vi "ConnectionTest.vi"() -> ()   [LabVIEW 2015]
uses:
  <vilib>/userdefined/High Color/IMAQdx.ctl
  <vilib>/vision/driver/IMAQdx.llb/IMAQdx Camera Control Mode.ctl
  <vilib>/vision/driver/IMAQdx.llb/IMAQdx Acquisition Mode.ctl
  <vilib>/vision/driver/IMAQdx.llb/IMAQdx Buffer Number Mode.ctl
  <vilib>/vision/driver/NI_Vision_Acquisition_Software.lvlib
panel:
  out "Image":T1(plugin-control)
  in  "Buffer Number Mode (Next)":T2
  in  "Number of Buffers":u32=1
  in  "Continuous?":T3
  out "error out":errorcluster
  in  "Camera Control Mode":T4
  in  "Session In":T5
  # "This is just me testing trying to connect the camera and LabView\n\nGenerally I will have a few programs titled testing where I am working on new things and then when they are complete or they have some functionality I go to Save As and do the thing where I rename the VI"
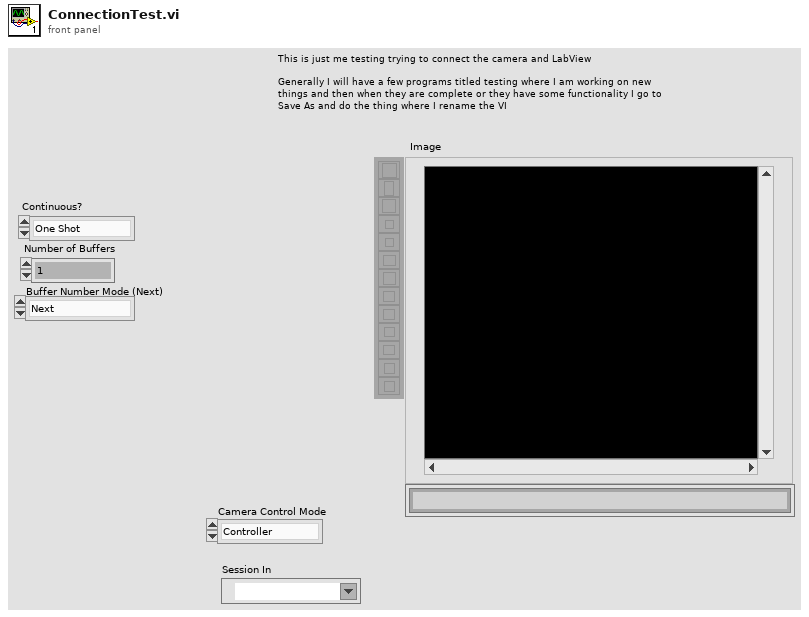
[diagram p1: front panel]
types:
  T1 = typedef "IMAQ Image.ctl" = refnum<image>
  T2 = typedef "NI_Vision_Acquisition_Software.lvlib/IMAQdx Buffer Number Mode.ctl" = enum32{"Next", "Last", "Buffer Number", "Every", "Last New"}
  T3 = typedef "NI_Vision_Acquisition_Software.lvlib/IMAQdx Acquisition Mode.ctl" = enum32{"One Shot", "Continuous"}
  T4 = typedef "NI_Vision_Acquisition_Software.lvlib/IMAQdx Camera Control Mode.ctl" = enum32{"Controller", "Listener"}
  T5 = typedef "IMAQdx.ctl" = refnum<k21>
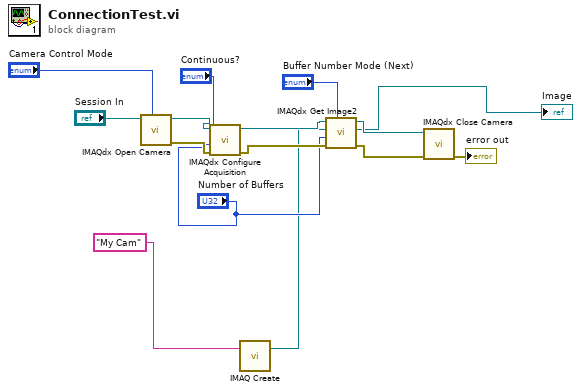
[diagram p0: block diagram]
diagram:
  n1 = call <vilib>:"IMAQdx Open Camera.vi"("Camera Control Mode"="Camera Control Mode", "Session In"="Session In") -> ("error out"=w11:errorcluster, "Session Out"=w12:T5)  [unwired: 8 in]
  n2 = call <vilib>:"IMAQdx Configure Acquisition.vi"("error in"=w11, "Number of Buffers"="Number of Buffers", "Continuous?"="Continuous?", "Session In"=w12) -> ("error out"=w8:errorcluster, "Session Out"=w9:T5)  [unwired: 6 in]
  n3 = call "IMAQ Create"("Image Name"="My Cam") -> ("New Image"=w4:T1)  [unwired: 4 in, 1 out]
  n4 = call <vilib>:"IMAQdx Get Image2.vi"("Buffer Number Mode (Next)"="Buffer Number Mode (Next)", "error in"=w8, "Buffer Number In"="Number of Buffers", "Image In"=w4, "Session In"=w9) -> ("error out"=w6:errorcluster, "Image Out"=→"Image":T1, "Session Out"=w7:T5)  [unwired: 3 in, 1 out]
  n5 = call <vilib>:"IMAQdx Close Camera.vi"("error in"=w6, "Session In"=w7) -> ("error out"=→"error out":errorcluster)  [unwired: 9 in]
